vi "SSC DAQmx Stop.vi"(0 "DAQmx SSC in":T1[](array[typedef]), 11 "error in":errorcluster) -> (4 "DAQmx SSC out":T1[](array[typedef]), 15 "error out":errorcluster)   [LabVIEW 2020]
doc: "Stops the tasks if any running."
uses:
  Pin Map/SSC DAQmx.ctl
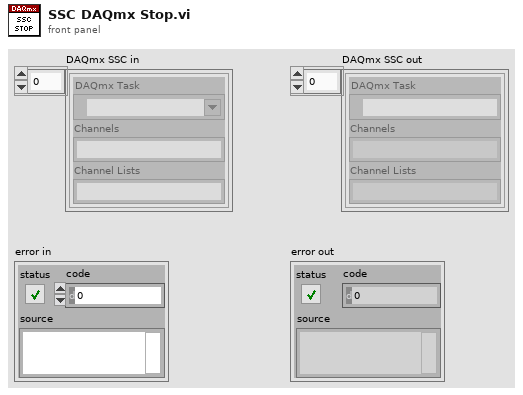
[diagram p1: front panel]
types:
  T1 = typedef "SSC DAQmx.ctl" = cluster{"DAQmx Task ":refnum<k21>, "Channels":string, "Channel Lists":string}
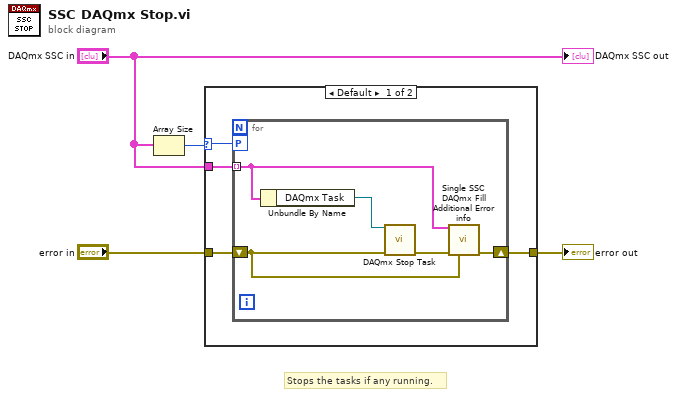
[diagram p0: block diagram]
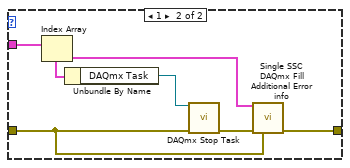
[diagram p2: hidden frame]
diagram:
  # "Stops the tasks if any running."
  n1 = Array Size(array="DAQmx SSC in") -> (size(s)=w2:i32)
  n2 = case shown="Default" w2 {
    selector: w2 -> [w6 _]
    tunnel: [w8 w18] -> w4
    tunnel: "error in" -> [w7 w16]
    tunnel: "DAQmx SSC in" -> [w5 w19]
    frame Default {
      n3 = for {
        tunnel: w5 -> [w10] mode=indexing
        workers-P: w6 -> [_]
        shift-right: [w13] -> w8
        shift-left: w7 -> [w12]
        n4 = Unbundle By Name(w10) -> ("DAQmx Task"=w9:refnum<k21>)
        n5 = call <vilib>:"DAQmx Stop Task.vi"("task/channels in"=w9, "error in"=w12) -> ("error out"=w11:errorcluster)  [unwired: 12 in, 1 out]
        n6 = call "Single SSC DAQmx Fill Additional Error info.vi"("DAQmx SSC in"=w10, "error in"=w11, "previous error in"=w12) -> ("error out"=w13:errorcluster)  [unwired: 12 in]
      }
    }
    frame 1 {
      n7 = Index Array(array=w19) -> (element=w14:T1)  [unwired: 1 in]
      n8 = Unbundle By Name(w14) -> ("DAQmx Task"=w17:refnum<k21>)
      n9 = call <vilib>:"DAQmx Stop Task.vi"("task/channels in"=w17, "error in"=w16) -> ("error out"=w15:errorcluster)  [unwired: 12 in, 1 out]
      n10 = call "Single SSC DAQmx Fill Additional Error info.vi"("DAQmx SSC in"=w14, "error in"=w15, "previous error in"=w16) -> ("error out"=w18:errorcluster)  [unwired: 12 in]
    }
  }
  "error out" <- w4
  "DAQmx SSC out" <- "DAQmx SSC in"
